vi "Label Targets3.vi"(8 "Score Threshold":dbl=75.0, 9 "Annotate":bool=TRUE, 10 "Targets":T2(array[cluster]), 11 "Image in":T1) -> (3 "Image out":T1)   [LabVIEW 2014]
doc: "Draw text scores near or on the particle. Scores above the threshold are green and underlined."
uses:
  <vilib>/vision/Image Controls.llb/IMAQ Image.ctl
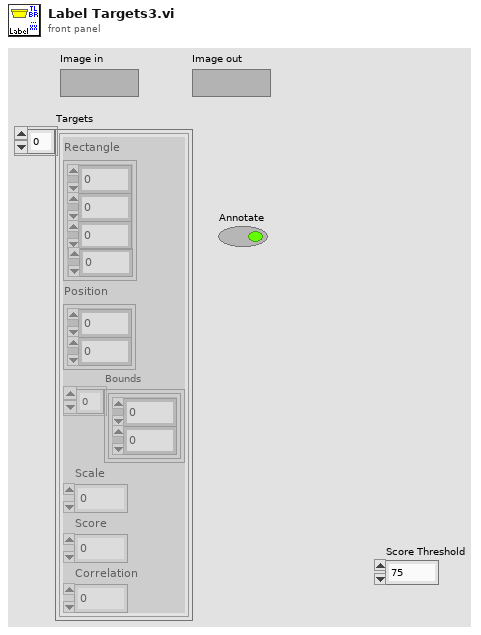
[diagram p1: front panel]
types:
  T1 = typedef "IMAQ Image.ctl" = refnum<image>
  T2 = cluster{"Rectangle":cluster{"Numeric":dbl, "Numeric 2":dbl, "Numeric 3":dbl, "Numeric 5":dbl}, "Position":cluster{"Numeric":dbl, "Numeric 2":dbl}, "Bounds":cluster{"Numeric":dbl, "Numeric 2":dbl}[], "Scale":dbl, "Score":dbl, "Correlation":dbl}[]
  T3 = cluster{"Desired Font (Application)":enum16{"User-specified Font", "Application Font", "System Font", "Dialog Font"}, "[User-specified Font]":cluster{"Font Name":string, "Size":i16, "Strikeout?":bool, "Italic?":bool, "Underline?":bool, "Outline?":bool, "Shadow?":bool, "Bold?":bool, "Rotation Angle":dbl}, "Horizontal Alignment":i16, "Vertical Alignment":i16}
  T4 = cluster{"Numeric":dbl, "Numeric 2":dbl, "Numeric 3":dbl, "Numeric 5":dbl}
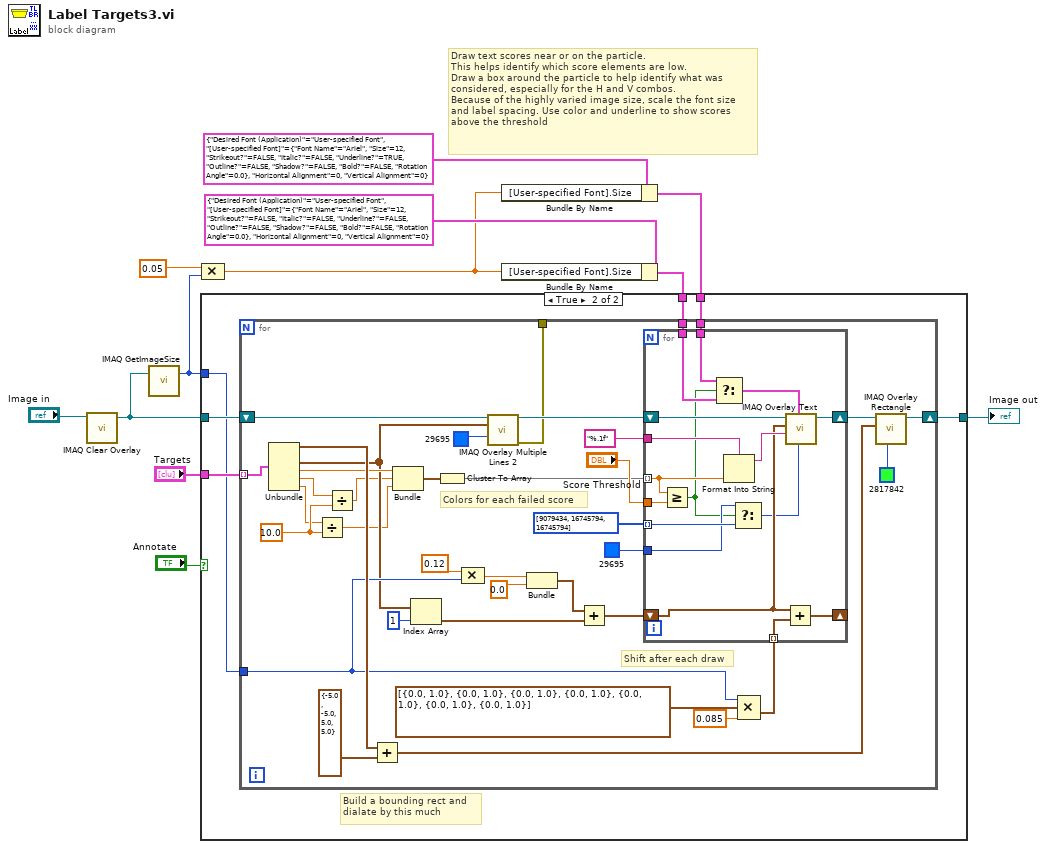
[diagram p0: block diagram]
diagram:
  # "Draw text scores near or on the particle.\nThis helps identify which score elements are low.\nDraw a box around the particle to help identify what was\nconsidered, especially for the H and V combos.\nBecause of the highly varied image size, scale the font size\nand label spacing. Use color and underline to show scores\nabove the threshold"
  n1 = call "IMAQ Clear Overlay"("Image"="Image in") -> ("Image Out"=w4:T1)  [unwired: 2 in, 8 out]
  n2 = call "IMAQ GetImageSize"("Image"=w4) -> ("Y Resolution"=w3:i32)  [unwired: 3 in, 2 out]
  n3 = Compound Arithmetic op=MULTIPLY(0.05, w3) -> (w2:dbl)
  n4 = Bundle By Name(cluster=T3 {"Desired Font (Application)"=enum."User-specified Font", "[User-specified Font]"={"Font Name"="Ariel", "Size"=12, "Strikeout?"=FALSE, "Italic?"=FALSE, "Underline?"=TRUE, "Outline?"=FALSE, "Shadow?"=FALSE, "Bold?"=FALSE, "Rotation Angle"=0.0}, "Horizontal Alignment"=0, "Vertical Alignment"=0} ("Font, Size & Style"), "[User-specified Font].Size"=w2) -> (w5:T3)
  n5 = Bundle By Name(cluster=T3 {"Desired Font (Application)"=enum."User-specified Font", "[User-specified Font]"={"Font Name"="Ariel", "Size"=12, "Strikeout?"=FALSE, "Italic?"=FALSE, "Underline?"=FALSE, "Outline?"=FALSE, "Shadow?"=FALSE, "Bold?"=FALSE, "Rotation Angle"=0.0}, "Horizontal Alignment"=0, "Vertical Alignment"=0} ("Font, Size & Style"), "[User-specified Font].Size"=w2) -> (w6:T3)
  n6 = case shown="True" "Annotate" {
    tunnel: [w13 w19] -> w12
    tunnel: "Targets" -> [_ w18]
    tunnel: w4 -> [w13 w17]
    tunnel: w5 -> [_ w16]
    tunnel: w6 -> [_ w15]
    tunnel: w3 -> [_ w14]
    frame False {
    }
    frame True {
      # "Build a bounding rect and\ndialate by this much"
      n7 = for {
        tunnel: w18 -> [w51] mode=indexing
        shift-right: [w52] -> w19
        shift-left: w17 -> [w32]
        tunnel: w14 -> [w34]
        tunnel: w16 -> [w39]
        tunnel: w15 -> [w38]
        tunnel: [w25] -> _
        w24 = 10.0
        # "Colors for each failed score"
        # "Shift after each draw"
        n8 = Unbundle(w51) -> ("Rectangle"=w48:T4, "Bounds"=w29:cluster{"Numeric":dbl, "Numeric 2":dbl}[], "Scale"=w46:dbl, "Score"=w21:dbl, "Correlation"=w22:dbl)  [unwired: 1 out]
        n9 = Divide(x=w22, y=w24) -> (x/y=w23:dbl)
        n10 = Divide(x=w21, y=w24) -> (x/y=w20:dbl)
        n11 = Add(x=w48, y=cluster{dbl, dbl, dbl, dbl} {-5.0, -5.0, 5.0, 5.0} ("output cluster")) -> (x+y=w50:cluster{dbl, dbl, dbl, dbl})
        n12 = Bundle("Scale"=w46, w20, w23) -> (w54:cluster{"Scale":dbl, dbl, dbl})  [unwired: 1 in]
        n13 = Index Array(array=w29, index=1) -> (element=w27:cluster{"Numeric":dbl, "Numeric 2":dbl})
        n14 = Cluster To Array(cluster=w54) -> (array=w47:dbl[])
        n15 = Compound Arithmetic op=MULTIPLY(0.12, w34) -> (w35:dbl)
        n16 = call "IMAQ Overlay Multiple Lines 2"("Image"=w32, "Line End Points"=w29, "Color"=u32 29695) -> ("Image Out"=w31:T1, "error out"=w25:errorcluster)  [unwired: 11 in]
        n17 = Bundle(w35, 0.0) -> (w37:cluster{dbl, dbl})  [unwired: 1 in]
        n18 = Add(x=w37, y=w27) -> (x+y=w56:cluster{dbl, dbl})
        n19 = Compound Arithmetic op=MULTIPLY(w34, cluster{dbl, dbl}[] [{0.0, 1.0}, {0.0, 1.0}, {0.0, 1.0}, {0.0, 1.0}, {0.0, 1.0}, {0.0, 1.0}, {0.0, 1.0}], 0.085) -> (w43:cluster{dbl, dbl}[])
        n20 = for {
          tunnel: w47 -> [w66] mode=indexing
          shift-right: [w69] -> _
          shift-left: w56 -> [w68]
          shift-right: [w70] -> w53
          shift-left: w31 -> [w71]
          tunnel: u32[] [9079434, 16745794, 16745794] -> [w67] mode=indexing
          tunnel: "Score Threshold" -> [w65]
          tunnel: w43 -> [w63] mode=indexing
          tunnel: "%.1f" ("format string") -> [w62]
          tunnel: u32 29695 ("Color") -> [w61]
          tunnel: w39 -> [w60]
          tunnel: w38 -> [w59]
          n21 = Greater Or Equal?(x=w66, y=w65) -> (x >= y?=w58:bool)
          n22 = Select(t=w60, s=w58, f=w59) -> (s? t:f=w57:T3)
          n23 = Format Into String(format string=w62, w66) -> (resulting string=w72:string)  [unwired: 2 in, 1 out]
          n24 = Select(t=w61, s=w58, f=w67) -> (s? t:f=w64:u32)
          n25 = Add(x=w63, y=w68) -> (x+y=w69:cluster{dbl, dbl})
          n26 = call "IMAQ Overlay Text"("Text Color (black)"=w64, "Font, Size & Style"=w57, "String"=w72, "Origin"=w68, "Image"=w71) -> ("Image Out"=w70:T1)  [unwired: 5 in, 1 out]
        }
        n27 = call "IMAQ Overlay Rectangle"("Color"=u32 2817842, "Rectangle"=w50, "Image"=w53) -> ("Image Out"=w52:T1)  [unwired: 7 in, 1 out]
      }
    }
  }
  "Image out" <- w12
